vi "Table Logging Setting.vi"(6 "length":i32=5, 7 "file path (dialog if empty)":path, 8 "error in (no error)":errorcluster, 9 "Logging Rate":T1, 10 "Data In":T2={"CommConnected_1"=FALSE, "Run_1?"=FALSE, "Fault_1?"=FALSE, "CommConnected_2"=FALSE, "Run_2?"=FALSE, "Fault_2?"=FALSE, "Motor Speed 2"=0.0, "Motor Speed_1"=28.0, "Motor Current_1"=0.0, "Motor Current_2"=0.0, "Motor1ConfigData"={"电机配置"=enum."配置1", "电压（V）"=0.0, "电流（A）"=0.0, "速度（RPM）"=0.0, "励磁方式"=enum."永磁"}, "Motor2ConfigData"={"电机配置"=enum."配置1", "电压（V）"=0.0, "电流（A）"=0.0, "速度（RPM）"=0.0, "励磁方式"=enum."永磁"}}, 11 "Record":bool) -> (0 "error out":errorcluster, 2 "Data Out":T2={"CommConnected_1"=FALSE, "Run_1?"=FALSE, "Fault_1?"=FALSE, "CommConnected_2"=FALSE, "Run_2?"=FALSE, "Fault_2?"=FALSE, "Motor Speed 2"=0.0, "Motor Speed_1"=28.0, "Motor Current_1"=0.0, "Motor Current_2"=0.0, "Motor1ConfigData"={"电机配置"=enum."配置1", "电压（V）"=0.0, "电流（A）"=0.0, "速度（RPM）"=0.0, "励磁方式"=enum."永磁"}, "Motor2ConfigData"={"电机配置"=enum."配置1", "电压（V）"=0.0, "电流（A）"=0.0, "速度（RPM）"=0.0, "励磁方式"=enum."永磁"}}, 3 "速度记录":string[][](table)=[["2018-04-13 14:46:04", "8.0", "0.0", "0.0", "0.0"], ["2018-04-13 14:46:05", "9.0", "0.0", "0.0", "0.0"], ["2018-04-13 14:46:06", "10.0", "0.0", "0.0", "0.0"], ["2018-04-13 14:46:07", "11.0", "0.0", "0.0", "0.0"], ["2018-04-13 14:46:08", "12.0", "0.0", "0.0", "0.0"], ["2018-04-13 14:46:09", "13.0", "0.0", "0.0", "0.0"], ["2018-04-13 14:46:10", "14.0", "0.0", "0.0", "0.0"], ["2018-04-13 14:46:11", "15.0", "0.0", "0.0", "0.0"], ["2018-04-13 14:46:13", "17.0", "0.0", "0.0", "0.0"], ["2018-04-13 14:46:15", "19.0", "0.0", "0.0", "0.0"], ["2018-04-13 14:46:17", "21.0", "0.0", "0.0", "0.0"], ["2018-04-13 14:46:48", "3.0", "0.0", "0.0", "0.0"], ["2018-04-13 14:46:50", "5.0", "0.0", "0.0", "0.0"], ["2018-04-13 14:46:52", "7.0", "0.0", "0.0", "0.0"], ["2018-04-13 14:46:54", "9.0", "0.0", "0.0", "0.0"], ["2018-04-13 14:46:58", "13.0", "0.0", "0.0", "0.0"], ["2018-04-13 14:47:02", "17.0", "0.0", "0.0", "0.0"], ["2018-04-13 14:47:06", "21.0", "0.0", "0.0", "0.0"], ["2018-04-13 14:47:10", "25.0", "0.0", "0.0", "0.0"]])   [LabVIEW 2018]
uses:
  Ctls/DisplayIndicator.ctl
  Ctls/MotroConfigData.ctl
  Ctls/MotorConfig.ctl
  Ctls/MagType.ctl
  Ctls/LoggingRate.ctl
  Ctls/DatabaseCmd.ctl
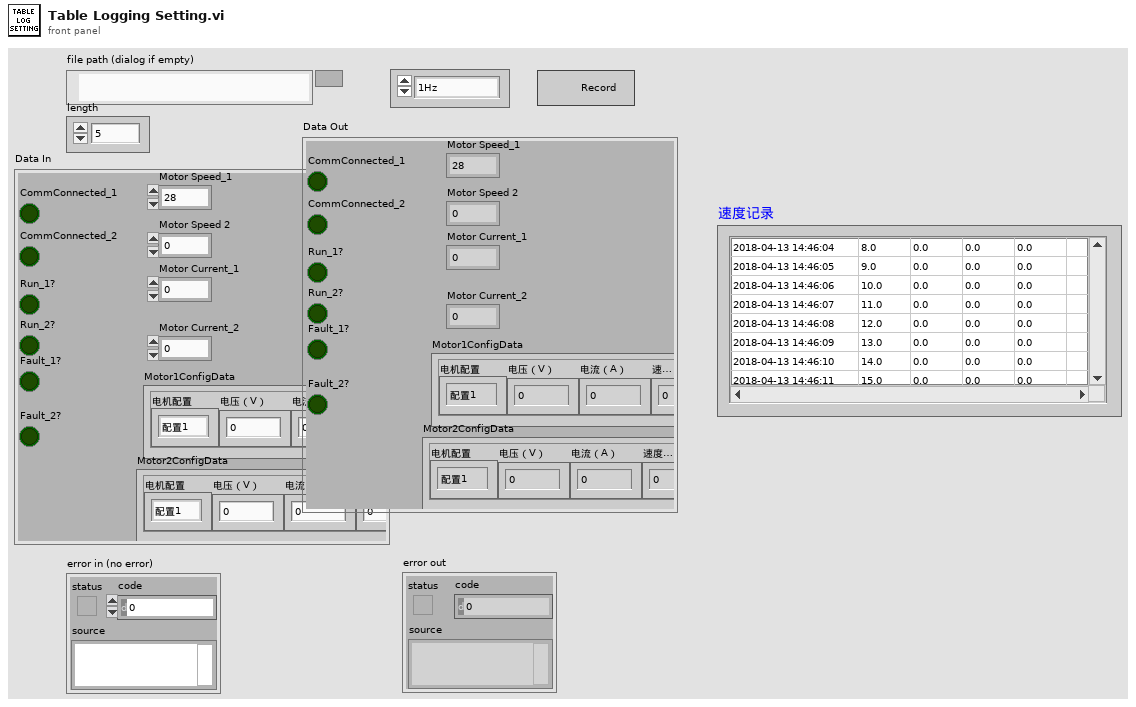
[diagram p1: front panel]
types:
  T1 = typedef "LoggingRate.ctl" = enum16{"1Hz", "2Hz", "5Hz", "10Hz"}
  T2 = typedef "DisplayIndicator.ctl" = cluster{"CommConnected_1":bool, "Run_1?":bool, "Fault_1?":bool, "CommConnected_2":bool, "Run_2?":bool, "Fault_2?":bool, "Motor Speed 2":sgl, "Motor Speed_1":sgl, "Motor Current_1":sgl, "Motor Current_2":sgl, "Motor1ConfigData":T3, "Motor2ConfigData":T3}
  T3 = typedef "MotroConfigData.ctl" = cluster{"电机配置":T4, "电压（V）":dbl, "电流（A）":dbl, "速度（RPM）":dbl, "励磁方式":T5}
  T4 = typedef "MotorConfig.ctl" = enum16{"配置1", "配置2", "配置3", "配置4"}
  T5 = typedef "MagType.ctl" = enum16{"永磁", "励磁"}
  T6 = typedef "DatabaseCmd.ctl" = enum16{"Insert Table Title", "Add One Record", "Delete Record", "Get Table Records", "Clear"}
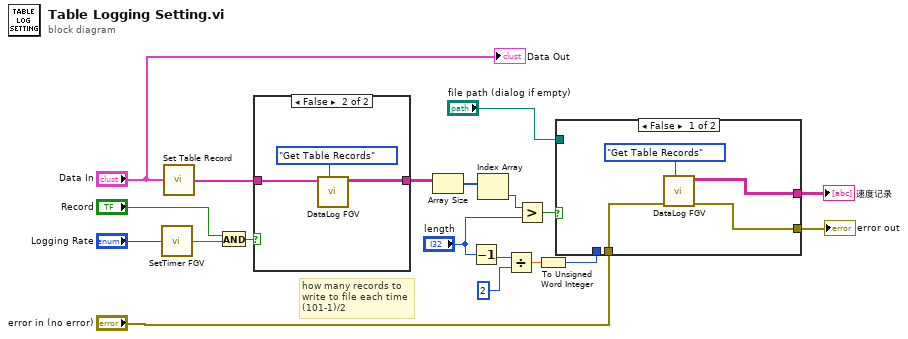
[diagram p0: block diagram]
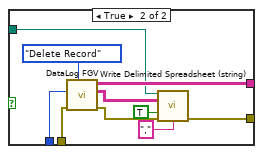
[diagram p2: hidden frame]
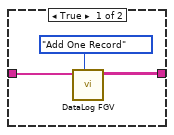
[diagram p3: hidden frame]
diagram:
  # "how many records to\nwrite to file each time\n(101-1)/2"
  n1 = call "SetTimer FGV.vi"("Logging Rate"="Logging Rate") -> ("Add?"=w16:bool)
  n2 = call "Set Table Record.vi"("Data In"="Data In") -> ("Record Out"=w18:string[])
  n3 = And(x="Record", y=w16) -> (x .and. y?=w15:bool)
  n4 = case shown="False" w15 {
    tunnel: w18 -> [w22 w25]
    tunnel: [w21 w24] -> w1
    frame True {
      n5 = call "DataLog FGV.vi"("Method"=DatabaseCmd."Add One Record", "New Record"=w22) -> ("速度记录"=w21:string[][])  [unwired: 7 in, 2 out]
    }
    frame False {
      n6 = call "DataLog FGV.vi"("Method"=DatabaseCmd."Get Table Records", "New Record"=w25) -> ("速度记录"=w24:string[][])  [unwired: 7 in, 2 out]
    }
  }
  n7 = Array Size(array=w1) -> (size(s)=w13:i32[])
  n8 = Decrement(x="length") -> (x-1=w9:i32)
  n9 = Index Array(array=w13) -> (element=w12:i32)  [unwired: 1 in]
  n10 = Divide(x=w9, y=2) -> (x/y=w7:dbl)
  n11 = Greater?(x=w12, y="length") -> (0:w11:bool)
  n12 = To Unsigned Word Integer(number=w7) -> (unsigned 16bit integer=w6:u16)
  n13 = case shown="False" w11 {
    tunnel: w6 -> [_ w39]
    tunnel: [w27 w37] -> w5
    tunnel: "error in (no error)" -> [w29 w34]
    tunnel: "file path (dialog if empty)" -> [_ w32]
    tunnel: [w26 w31] -> w2
    frame False {
      n14 = call "DataLog FGV.vi"("Method"=DatabaseCmd."Get Table Records", "error in (no error)"=w29) -> ("error out"=w26:errorcluster, "速度记录"=w27:string[][])  [unwired: 7 in, 1 out]
    }
    frame True {
      n15 = call "DataLog FGV.vi"("Method"=DatabaseCmd."Delete Record", "error in (no error)"=w34, "length"=w39) -> ("error out"=w35:errorcluster, "log to file"=w36:string[][], "速度记录"=w37:string[][])  [unwired: 6 in]
      n16 = call "Write Delimited Spreadsheet (string).vi"("Path"=w32, "2D data"=w36, "append to file?"=TRUE ("append to file? (new file:F)"), "error in"=w35, "delimiter (\\t)"="," ("delimiter (\\t)")) -> ("error out"=w31:errorcluster)  [unwired: 9 in, 1 out]
    }
  }
  "速度记录" <- w5
  "error out" <- w2
  "Data Out" <- "Data In"
